vi "SetConfig.vi"(8 "error in (no error)":errorcluster, 10 "Variant":variant, 11 "StateFunction in":refnum<class "StateFunction.lvclass">) -> (0 "error out":errorcluster, 3 "StateFunction out":refnum<class "StateFunction.lvclass">)   [LabVIEW 2014, in "StateFunction.lvclass"]
uses:
  StateFunction.lvclass
  Typedef/StateConfig.ctl
  ArbitraryFunction/TypeDefs/Arbitrary.ctl
  StateFunction.lvclass/StateFunction.ctl
  ArbitraryFunction/ArbitraryFunction.lvclass/ArbitraryFunction.ctl
  Accessors/Write X.vi
  Accessors/Write A.vi
  Accessors/Write B.vi
  Accessors/Write C.vi
  Accessors/Write D.vi
  ArbitraryFunction/Accessors/Write Arbs.vi
  ArbitraryFunction/ArbitraryFunction.lvclass
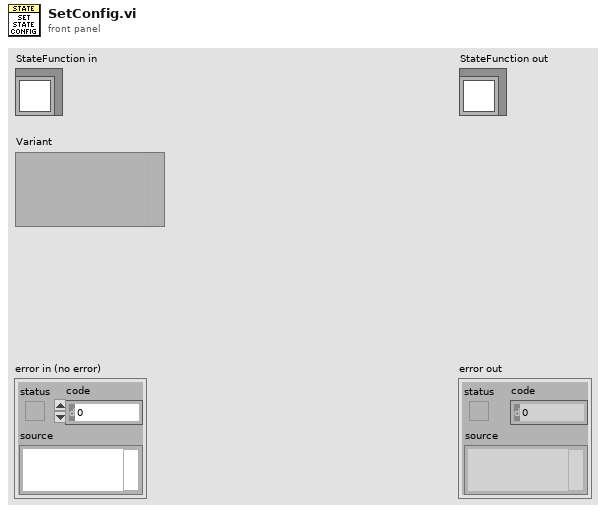
[diagram p1: front panel]
types:
  T1 = typedef "StateFunction.lvclass/StateConfig.ctl" = cluster{"X":dbl[][], "ConfigX":bool, "A":dbl[][][], "ConfigA":bool, "B":dbl[][], "ConfigB":bool, "C":dbl[][][], "ConfigC":bool, "D":dbl[][], "ConfigD":bool, "ARBs":T2[], "ConfigArbs":bool}
  T2 = typedef "Functions.lvlib/ArbitraryFunction.lvclass/Arbitrary.ctl" = cluster{"Handle":string, "Size":i32, "Gain":dbl, "Offset":dbl, "Waveform":waveform(dbl)}
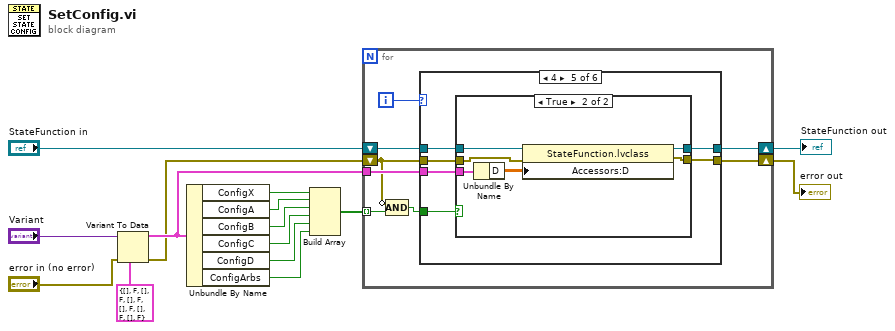
[diagram p0: block diagram]
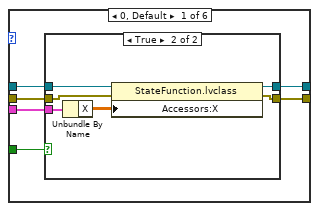
[diagram p2: hidden frame]
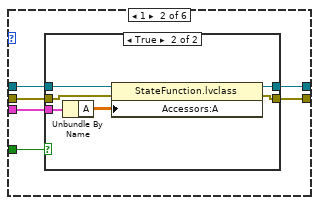
[diagram p4: hidden frame]
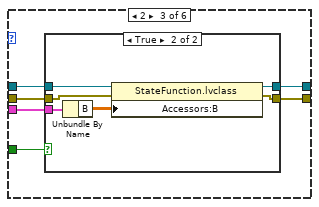
[diagram p6: hidden frame]
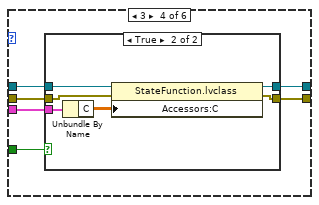
[diagram p8: hidden frame]
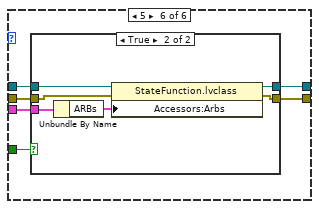
[diagram p11: hidden frame]
diagram:
  n1 = Variant To Data(error in="error in (no error)", type=T1 {"X"=[], "ConfigX"=FALSE, "A"=[], "ConfigA"=FALSE, "B"=[], "ConfigB"=FALSE, "C"=[], "ConfigC"=FALSE, "D"=[], "ConfigD"=FALSE, "ARBs"=[], "ConfigArbs"=FALSE} ("StateConfig"), Variant="Variant") -> (data=w4:T1, error out=w2:errorcluster)
  n2 = Unbundle By Name(w4) -> ("ConfigX"=w12:bool, "ConfigA"=w11:bool, "ConfigB"=w10:bool, "ConfigC"=w9:bool, "ConfigD"=w8:bool, "ConfigArbs"=w7:bool)
  n3 = Build Array(w12, w11, w10, w9, w8, w7) -> (w6:bool[])
  n4 = for {
    tunnel: w6 -> [w17] mode=indexing
    shift-right: [w22] -> w3
    shift-left: "StateFunction in" -> [w21]
    tunnel: w4 -> [w20]
    shift-right: [w19] -> w1
    shift-left: w2 -> [w16]
    i -> [w23]
    n5 = Compound Arithmetic op=AND(invert w16, w17) -> (w18:bool)
    n6 = case shown="4" w23 {
      tunnel: w18 -> [w29 w43 w57 w71 w85 w99]
      tunnel: [w28 w42 w56 w70 w84 w98] -> w22
      tunnel: w21 -> [w27 w41 w55 w69 w83 w97]
      tunnel: w20 -> [w26 w40 w54 w68 w82 w96]
      tunnel: w16 -> [w25 w39 w53 w67 w81 w95]
      tunnel: [w24 w38 w52 w66 w80 w94] -> w19
      frame 0, Default {
        n7 = case shown="True" w29 {
          tunnel: [w31 w36] -> w28
          tunnel: w27 -> [w31 w37]
          tunnel: w26 -> [_ w35]
          tunnel: w25 -> [w30 w33]
          tunnel: [w30 w32] -> w24
          frame False {
          }
          frame True {
            n8 = Unbundle By Name(w35) -> ("X"=w34:dbl[][])
            n9 = property class="StateFunction.lvclass"(reference=w37, error in=w33, "Accessors:X"=w34) -> (reference out=w36:refnum<class "StateFunction.lvclass">, error out=w32:errorcluster)
          }
        }
      }
      frame 1 {
        n10 = case shown="True" w43 {
          tunnel: [w45 w50] -> w42
          tunnel: w41 -> [w45 w51]
          tunnel: w40 -> [_ w49]
          tunnel: w39 -> [w44 w47]
          tunnel: [w44 w46] -> w38
          frame False {
          }
          frame True {
            n11 = Unbundle By Name(w49) -> ("A"=w48:dbl[][][])
            n12 = property class="StateFunction.lvclass"(reference=w51, error in=w47, "Accessors:A"=w48) -> (reference out=w50:refnum<class "StateFunction.lvclass">, error out=w46:errorcluster)
          }
        }
      }
      frame 2 {
        n13 = case shown="True" w57 {
          tunnel: [w59 w64] -> w56
          tunnel: w55 -> [w59 w65]
          tunnel: w54 -> [_ w63]
          tunnel: w53 -> [w58 w61]
          tunnel: [w58 w60] -> w52
          frame False {
          }
          frame True {
            n14 = Unbundle By Name(w63) -> ("B"=w62:dbl[][])
            n15 = property class="StateFunction.lvclass"(reference=w65, error in=w61, "Accessors:B"=w62) -> (reference out=w64:refnum<class "StateFunction.lvclass">, error out=w60:errorcluster)
          }
        }
      }
      frame 3 {
        n16 = case shown="True" w71 {
          tunnel: [w73 w78] -> w70
          tunnel: w69 -> [w73 w79]
          tunnel: w68 -> [_ w77]
          tunnel: w67 -> [w72 w75]
          tunnel: [w72 w74] -> w66
          frame False {
          }
          frame True {
            n17 = Unbundle By Name(w77) -> ("C"=w76:dbl[][][])
            n18 = property class="StateFunction.lvclass"(reference=w79, error in=w75, "Accessors:C"=w76) -> (reference out=w78:refnum<class "StateFunction.lvclass">, error out=w74:errorcluster)
          }
        }
      }
      frame 4 {
        n19 = case shown="True" w85 {
          tunnel: [w87 w92] -> w84
          tunnel: w83 -> [w87 w93]
          tunnel: w82 -> [_ w91]
          tunnel: w81 -> [w86 w89]
          tunnel: [w86 w88] -> w80
          frame False {
          }
          frame True {
            n20 = Unbundle By Name(w91) -> ("D"=w90:dbl[][])
            n21 = property class="StateFunction.lvclass"(reference=w93, error in=w89, "Accessors:D"=w90) -> (reference out=w92:refnum<class "StateFunction.lvclass">, error out=w88:errorcluster)
          }
        }
      }
      frame 5 {
        n22 = case shown="True" w99 {
          tunnel: [w101 w106] -> w98
          tunnel: w97 -> [w101 w107]
          tunnel: w96 -> [_ w105]
          tunnel: w95 -> [w100 w103]
          tunnel: [w100 w102] -> w94
          frame False {
          }
          frame True {
            n23 = Unbundle By Name(w105) -> ("ARBs"=w104:T2[])
            n24 = property class="StateFunction.lvclass"(reference=w107, error in=w103, "Accessors:Arbs"=w104) -> (reference out=w106:refnum<class "StateFunction.lvclass">, error out=w102:errorcluster)
          }
        }
      }
    }
  }
  "error out" <- w1
  "StateFunction out" <- w3
